vi "Calculate Throughput.vi"(4 "FPGA FIFO clock":dbl format="%#_6p", 6 "bytes per element":u64, 8 "transfer count":u64, 9 "previous transfer count":u64, 10 "iteration count":u64, 11 "previous iteration count":u64) -> (3 "throughput (B/s)":dbl format="%#_6p")   [LabVIEW 2013]
doc: "This SubVI calculates throughput in Bytes per second (B/s) based on the number of transfers, the number of loop iterations, the number of bytes per element and the clock rate of the FPGA SCTL."
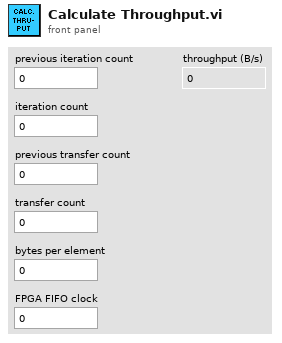
[diagram p1: front panel]
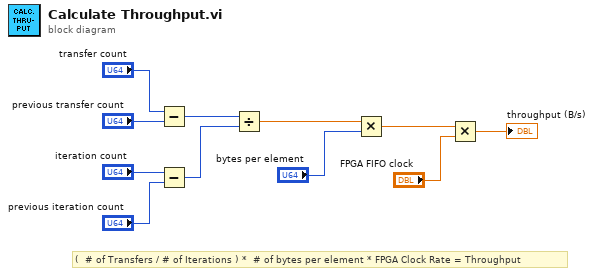
[diagram p0: block diagram]
diagram:
  # "(  # of Transfers / # of Iterations ) *  # of bytes per element * FPGA Clock Rate = Throughput"
  n1 = Subtract(x="transfer count", y="previous transfer count") -> (x-y=w3:u64)
  n2 = Subtract(x="iteration count", y="previous iteration count") -> (x-y=w4:u64)
  n3 = Divide(x=w3, y=w4) -> (x/y=w5:dbl)
  n4 = Multiply(x=w5, y="bytes per element") -> (x*y=w6:dbl)
  n5 = Multiply(x=w6, y="FPGA FIFO clock") -> (x*y=→"throughput (B/s)":dbl)
